vi "SendActorCoreMsg.vi"(8 "error in (no error)":errorcluster, 9 "Data":variant, 10 "Msg":T1, 11 "PLC_Module in":refnum<class "PLC_Module.lvclass">) -> (0 "error out":errorcluster, 3 "PLC_Module out":refnum<class "PLC_Module.lvclass">)   [LabVIEW 2025, in "PLC_Module.lvlib" / "PLC_Module.lvclass"]
uses:
  PLC_Module.lvclass
  PLC_Module.lvclass/PLC_Module.ctl
  Msg&Data.ctl
  Msg.ctl
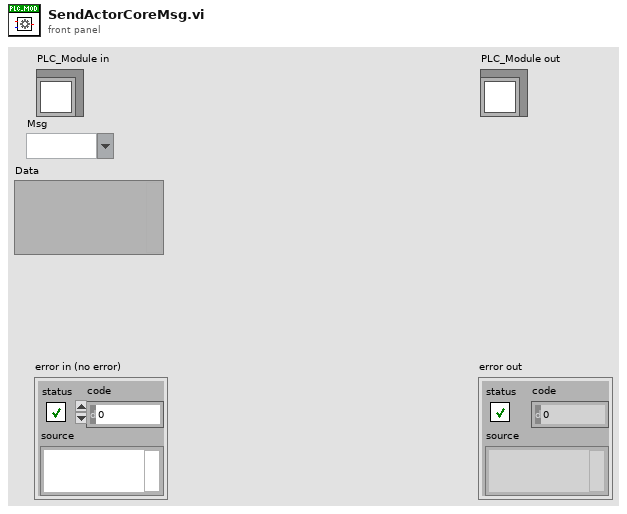
[diagram p1: front panel]
types:
  T1 = typedef "Msg.ctl" = string
  T2 = typedef "Msg&Data.ctl" = cluster{"Msg":T1, "Data":variant}
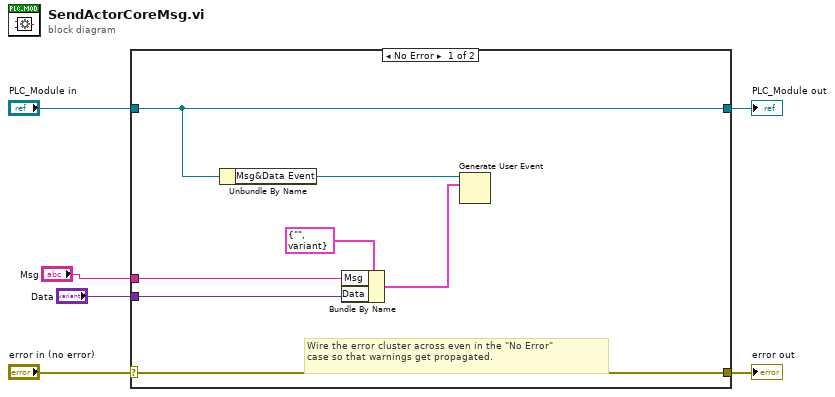
[diagram p0: block diagram]
diagram:
  n1 = case shown="No Error" "error in (no error)" {
    selector: "error in (no error)" -> [w13 w15]
    tunnel: [w13 w15] -> w5
    tunnel: [w12 w14] -> w3
    tunnel: "PLC_Module in" -> [w12 w14]
    tunnel: "Data" -> [w8 _]
    tunnel: "Msg" -> [w7 _]
    frame No Error {
      # "Wire the error cluster across even in the \"No Error\"\ncase so that warnings get propagated."
      n2 = Unbundle By Name(w12) -> ("Msg&Data Event"=w11:refnum<user-event>)
      n3 = Bundle By Name(cluster=T2 {"Msg"="", "Data"=variant} ("Msg&Data"), "Msg"=w7, "Data"=w8) -> (w9:T2)
      n4 = Generate User Event(user event=w11, event data cluster=w9) -> ()  [unwired: 2 in, 2 out]
    }
    frame Error {
    }
  }
  "error out" <- w5
  "PLC_Module out" <- w3
